vi "getTimeStamp.vi"(8 "error in (no error)":errorcluster, 11 "SALCommunicatorTC in":refnum<class "SALCommunicatorTC.lvclass">) -> (0 "error out":errorcluster, 2 "timestamp":dbl, 3 "SALCommunicatorTC out":refnum<class "SALCommunicatorTC.lvclass">)   [LabVIEW 2016, in "SALCommunicatorTC.lvclass"]
uses:
  SALCommunicatorTC.lvclass
  ts_sallv_exa/SALLV_EXA.lvlib
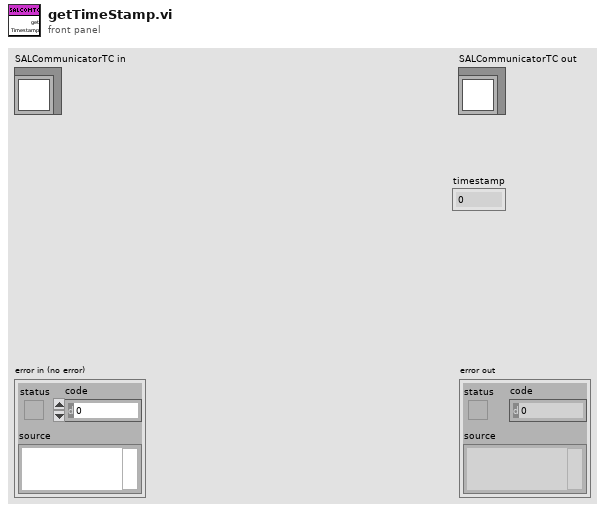
[diagram p1: front panel]
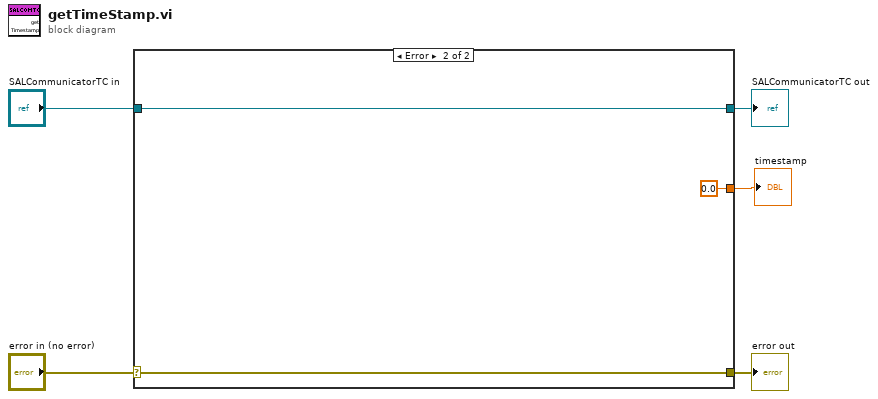
[diagram p0: block diagram]
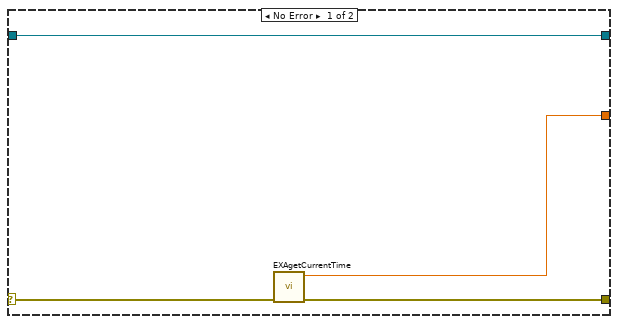
[diagram p2: hidden frame]
diagram:
  n1 = case shown="Error" "error in (no error)" {
    selector: "error in (no error)" -> [w8 w12]
    tunnel: [w7 w12] -> w4
    tunnel: [w9 w11] -> w2
    tunnel: "SALCommunicatorTC in" -> [w9 w11]
    tunnel: [w6 0.0 ("function return")] -> w1
    frame No Error {
      n2 = call "EXAgetCurrentTime.vi"("error in (no error)"=w8) -> ("error out"=w7:errorcluster, "function return"=w6:dbl)  [unwired: 9 in]
    }
    frame Error {
    }
  }
  "error out" <- w4
  "SALCommunicatorTC out" <- w2
  "timestamp" <- w1
